vi "Accumulated Correlation HPRF 3D.vi"(5 "Ntheta":i32=16, 6 "Sensor Locations (cm, cm, cm)":dbl[][](array[numeric])=[[0.0, 0.0, -5.08], [11.43, 0.0, 0.0], [0.0, 11.43, 0.0], [-11.43, 0.0, 0.0], [0.0, -11.43, 0.0], [0.0, 0.0, 5.08]], 7 "Nr":i32=16, 8 "Sound Velocity (cm/s)":dbl=576000.0, 9 "Sampling Rate":i32=500000, 11 "Waveforms":dbl[][](array[numeric])) -> (2 "Coordinates (cm, cm, cm)":cluster{"x":dbl, "y":dbl, "z":dbl})   [LabVIEW 2013]
uses:
  <vilib>/Analysis/2dsp.llb/1D Cross Correlation (DBL).vi
  <vilib>/Analysis/NI_AALPro.lvlib
panel:
  out "theta":dbl
  out "r":dbl
  out "Waveform Graph":dbl[][](graph)
  out "Lag Matrix":dbl[][](array[numeric])
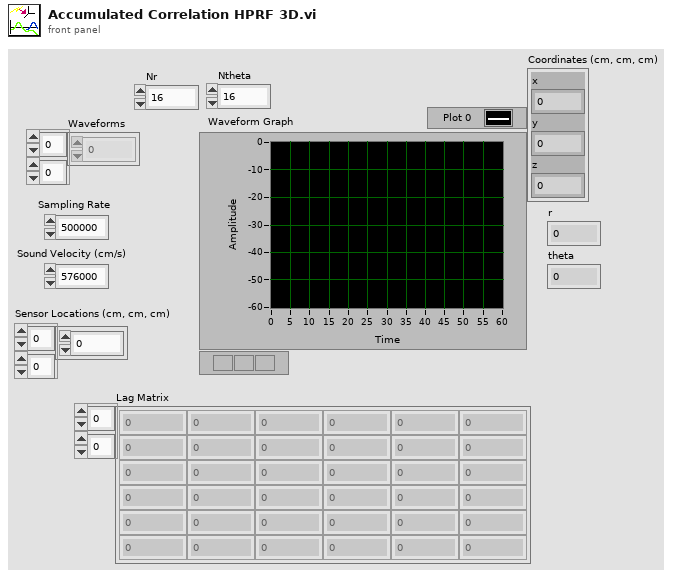
[diagram p1: front panel]
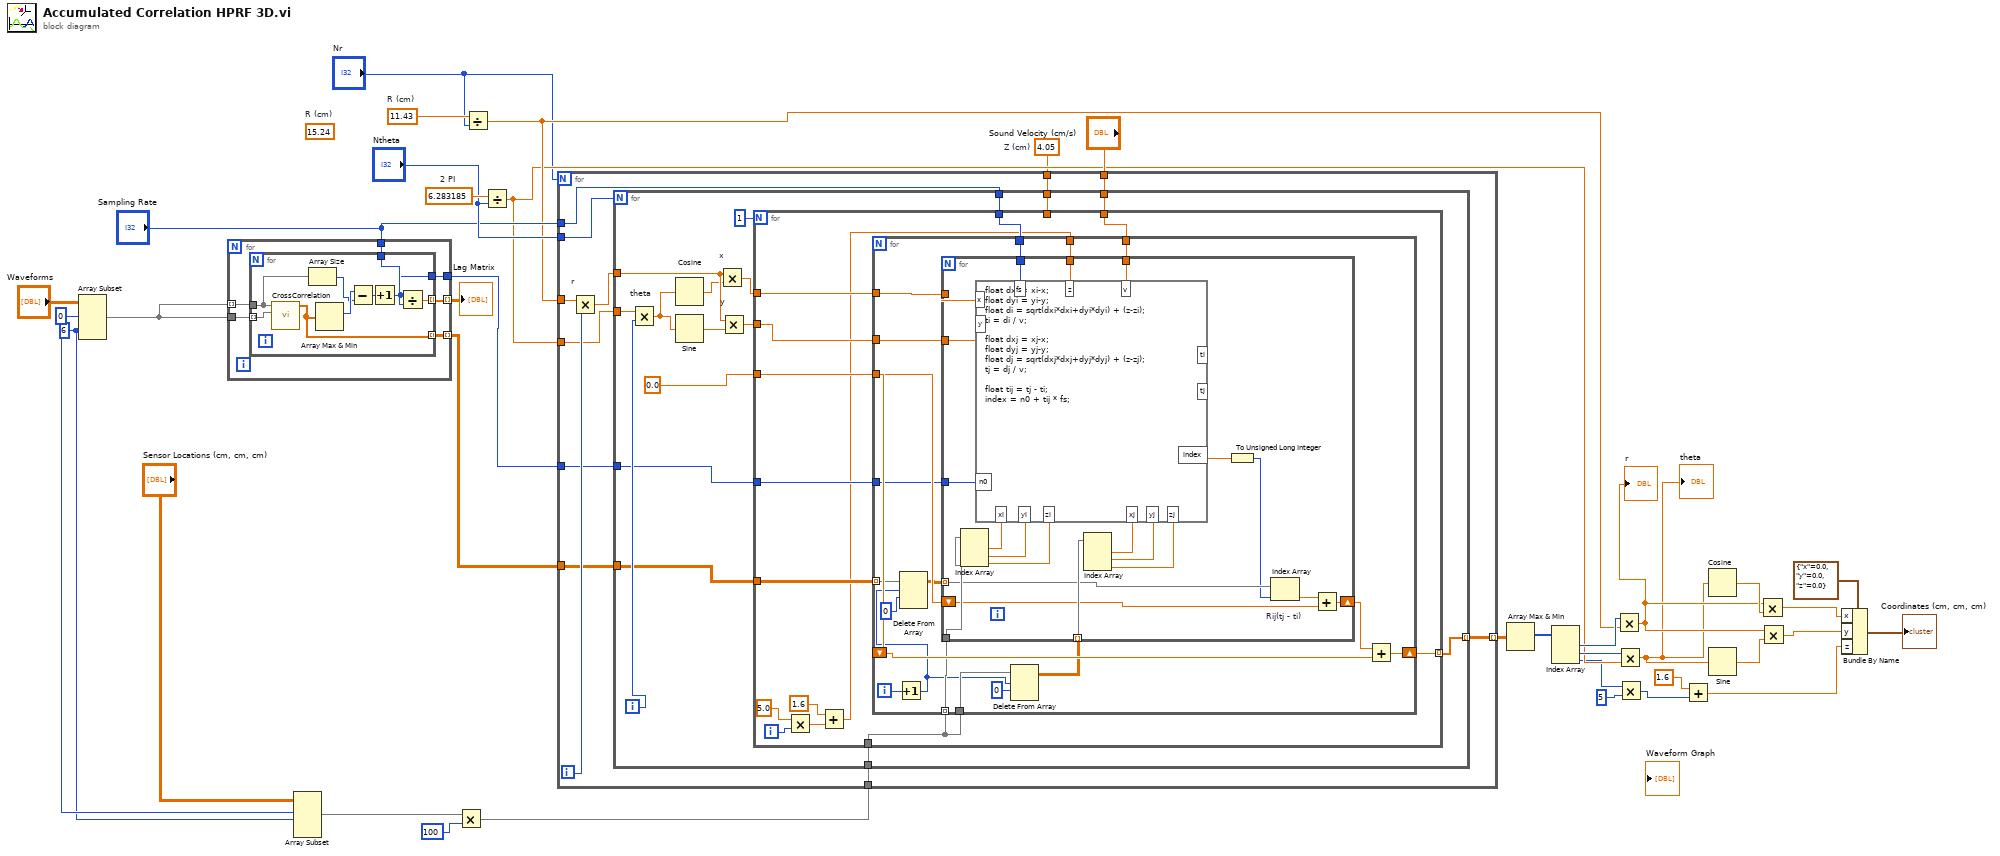
[diagram p0: block diagram]
diagram:
  (unwired) 15.24  # R (cm)
  w9 = 6 ("length")
  w10 = 0 ("index")
  w36 = 11.43  # R (cm)
  w35 = 6.283185  # 2 PI
  w16 = 4.05  # Z (cm)
  n1 = Array Subset(array="Waveforms", index (row)=w10, length (row)=w9) -> (w13:dbl[][])  [unwired: 2 in]
  n2 = for {
    tunnel: w13 -> [w42] mode=indexing
    tunnel: w13 -> [w43]
    tunnel: "Sampling Rate" -> [w41]
    tunnel: [w40] -> w37 mode=indexing
    tunnel: [w39] -> w30 mode=indexing
    tunnel: [w38] -> w31
    n3 = for {
      tunnel: w43 -> [w52] mode=indexing
      tunnel: w42 -> [w51]
      tunnel: w41 -> [w49]
      tunnel: [w48] -> w40 mode=indexing
      tunnel: [w46] -> w39 mode=indexing
      tunnel: [w44] -> w38
      n4 = call-poly <vilib>:"CrossCorrelation.vi"("Y"=w52, "X"=w51) -> ("Rxy"=w46:dbl[])  [unwired: 8 in, 1 out]
      n5 = Array Size(array=w51) -> (size(s)=w45:i32)
      n6 = Array Max & Min(array=w46) -> (max index (indices)=w50:i32)  [unwired: 3 out]
      n7 = Subtract(x=w50, y=w45) -> (x-y=w47:i32)
      n8 = Increment(x=w47) -> (x+1=w44:i32)
      n9 = Divide(x=w44, y=w49) -> (x/y=w48:dbl)
    }
  }
  "Lag Matrix" <- w37
  n10 = Array Subset(array="Sensor Locations (cm, cm, cm)", index (row)=w10, length (row)=w9) -> (w11:dbl[][])  [unwired: 2 in]
  n11 = Multiply(x=w11, y=100) -> (x*y=w28:dbl[][])
  n12 = Divide(x=w36, y="Nr") -> (x/y=w24:dbl)
  n13 = Divide(x=w35, y="Ntheta") -> (x/y=w23:dbl)
  n14 = for {
    N: "Nr" -> [_]
    tunnel: [w64] -> w8 mode=indexing
    tunnel: "Ntheta" -> [w63]
    tunnel: w24 -> [w62]
    tunnel: w23 -> [w60]
    tunnel: w28 -> [w59]
    tunnel: w16 -> [w58]
    tunnel: "Sound Velocity (cm/s)" -> [w57]
    tunnel: "Sampling Rate" -> [w56]
    tunnel: w31 -> [w55]
    tunnel: w30 -> [w54]
    i -> [w61]
    n15 = Multiply "r"(x=w62, y=w61) -> (x*y=w53:dbl)
    n16 = for {
      N: w63 -> [_]
      tunnel: [w80] -> w64 mode=indexing
      tunnel: w60 -> [w79]
      tunnel: w53 -> [w77]
      tunnel: w59 -> [w74]
      tunnel: w58 -> [w73]
      tunnel: w57 -> [w72]
      tunnel: w56 -> [w71]
      tunnel: w55 -> [w70]
      tunnel: w54 -> [w69]
      i -> [w78]
      n17 = Multiply "theta"(x=w79, y=w78) -> (x*y=w68:dbl)
      n18 = Cosine(x=w68) -> (cos(x)=w76:dbl)
      n19 = Sine(x=w68) -> (sin(x)=w75:dbl)
      n20 = Multiply "x"(x=w77, y=w76) -> (x*y=w67:dbl)
      n21 = Multiply "y"(x=w77, y=w75) -> (x*y=w66:dbl)
      n22 = for {
        N: 1 -> [_]
        tunnel: 0.0 -> [w95]
        tunnel: [w94] -> w80 mode=indexing
        tunnel: w74 -> [w93]
        tunnel: w73 -> [_]
        tunnel: w72 -> [w92]
        tunnel: w71 -> [w91]
        tunnel: w70 -> [w90]
        tunnel: w69 -> [w89]
        tunnel: w67 -> [w88]
        tunnel: w66 -> [w87]
        i -> [w86]
        n23 = Multiply(x=5.0, y=w86) -> (x*y=w85:dbl)
        n24 = Add(x=1.6, y=w85) -> (x+y=w83:dbl)
        n25 = for {
          shift-right: [w111] -> w94
          shift-left: w95 -> [w112]
          tunnel: w95 -> [w114]
          tunnel: w88 -> [w110]
          tunnel: w87 -> [w109]
          tunnel: w93 -> [w108] mode=indexing
          tunnel: w93 -> [w102]
          tunnel: w83 -> [w107]
          tunnel: w92 -> [w106]
          tunnel: w91 -> [w105]
          tunnel: w90 -> [w104]
          tunnel: w89 -> [w99] mode=indexing
          i -> [w103]
          n26 = Increment(x=w103) -> (x+1=w96:i32)
          n27 = Delete From Array(array=w99, length=w96, index (row)=0) -> (array with subset deleted=w98:dbl[][])  [unwired: 1 in, 1 out]
          n28 = Delete From Array(array=w102, length=w96, index (row)=0) -> (array with subset deleted=w100:dbl[][])  [unwired: 1 in, 1 out]
          n29 = for {
            shift-right: [w119] -> w113
            shift-left: w114 -> [w117]
            tunnel: w110 -> [w130]
            tunnel: w109 -> [w129]
            tunnel: w100 -> [w133] mode=indexing
            tunnel: w108 -> [w134]
            tunnel: w107 -> [w132]
            tunnel: w106 -> [w131]
            tunnel: w105 -> [w124]
            tunnel: w104 -> [w123]
            tunnel: w98 -> [w121] mode=indexing
            n30 = Index Array(array=w134) -> (element #1=w128:dbl, element #2=w127:dbl, element #3=w116:dbl)  [unwired: 3 in]
            n31 = Index Array(array=w133) -> (element #1=w126:dbl, element #2=w125:dbl, element #3=w115:dbl)  [unwired: 3 in]
            n32 = formula code="float dxi = xi-x;\nfloat dyi = yi-y;\nfloat di = sqrt(dxi*dxi+dyi*dyi) + (z-zi);\nti = di / v;\n\nfloat dxj = xj-x;\nfloat dyj = yj-y;\nfloat dj = sqrt(dxj*dxj+dyj*dyj) + (z-zj);\ntj = dj / v;\n\nfloat tij = tj - ti;\nindex = n0 + tij * fs;"("xi"=w128, "yi"=w127, "xj"=w126, "yj"=w125, "x"=w130, "y"=w129, "z"=w132, "v"=w131, "fs"=w124, "n0"=w123, "zi"=w116, "zj"=w115) -> ("index"=w122:dbl)  [unwired: 2 out]
            n33 = To Unsigned Long Integer(number=w122) -> (unsigned 32bit integer=w120:u32)
            n34 = Index Array "Rij(tj - ti)"(array=w121, index=w120) -> (element=w118:dbl)
            n35 = Add(x=w118, y=w117) -> (x+y=w119:dbl)
          }
          n36 = Add(x=w113, y=w112) -> (x+y=w111:dbl)
        }
      }
    }
  }
  n37 = Array Max & Min(array=w8) -> (max index (indices)=w27:i32[])  [unwired: 3 out]
  n38 = Index Array(array=w27) -> (element #1=w26:i32, element #2=w25:i32, element #3=w6:i32)  [unwired: 3 in]
  n39 = Multiply(x=w26, y=w24) -> (x*y=w20:dbl)
  "r" <- w20
  n40 = Multiply(x=w25, y=w23) -> (x*y=w19:dbl)
  "theta" <- w19
  n41 = Multiply(x=w6, y=5) -> (x*y=w4:i32)
  n42 = Add(x=1.6, y=w4) -> (x+y=w3:dbl)
  n43 = Cosine(x=w19) -> (cos(x)=w22:dbl)
  n44 = Sine(x=w19) -> (sin(x)=w21:dbl)
  n45 = Multiply ("x*y")(x=w20, y=w22) -> (x*y=w18:dbl)
  n46 = Multiply ("x*y")(x=w20, y=w21) -> (x*y=w17:dbl)
  n47 = Bundle By Name(cluster=cluster{"x":dbl, "y":dbl, "z":dbl} {"x"=0.0, "y"=0.0, "z"=0.0} ("input cluster"), "x"=w18, "y"=w17, "z"=w3) -> (→"Coordinates (cm, cm, cm)":cluster{"x":dbl, "y":dbl, "z":dbl})
